vi "Add to Array.vi"(8 "error in (no error)":errorcluster, 9 "Module?":bool, 10 "Position Index":dbl, 11 "Database Entry in":refnum<class "Database Entry.lvclass">) -> (0 "error out":errorcluster, 3 "Database Entry out":refnum<class "Database Entry.lvclass">)   [LabVIEW 2021, in "Database Entry.lvclass"]
uses:
  Database Entry.lvclass
  Stack/Stack.lvclass
  Database Entry.lvclass/Database Entry.ctl
panel:
  out "Array":dbl[](array[numeric])
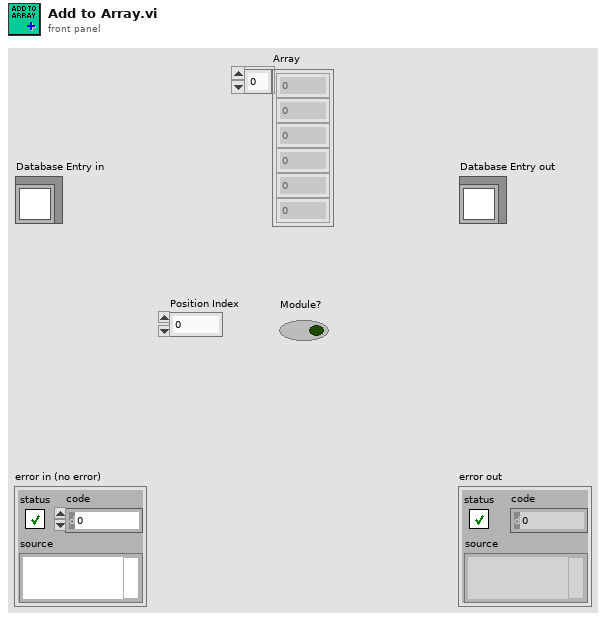
[diagram p1: front panel]
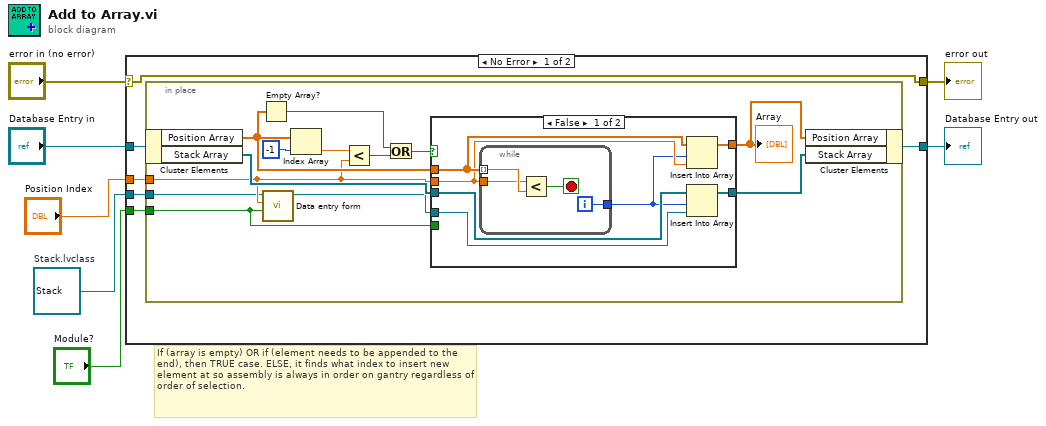
[diagram p0: block diagram]
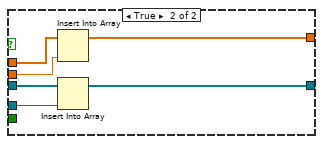
[diagram p2: hidden frame]
diagram:
  w2 = refnum<class "Stack.lvclass"> refnum  # Stack.lvclass
  # "If (array is empty) OR if (element needs to be appended to the end), then TRUE case. ELSE, it finds what index to insert new element at so assembly is always in order on gantry regardless of order of selection."
  n1 = case shown="No Error" "error in (no error)" {
    selector: "error in (no error)" -> [w13 w45]
    tunnel: [w13 w45] -> w6
    tunnel: [w10 w44] -> w4
    tunnel: "Database Entry in" -> [w11 w44]
    tunnel: w2 -> [w12 _]
    tunnel: "Position Index" -> [w9 _]
    tunnel: "Module?" -> [w8 _]
    frame No Error {
      n2 = in-place {
        in-place-border: w12 -> [w14]
        in-place-border: w9 -> [w16]
        in-place-border: w8 -> [w15]
        n3 = in-place-cluster #1(w11) -> ("Position Array"=w23:dbl[], "Stack Array"=w26:refnum<class "Stack.lvclass">[])
        n4 = Empty Array?(array=w23) -> (empty?=w20:bool)
        n5 = call "Data entry form.vi"("Module?"=w15, "Position"=w16, "Stack in"=w14) -> ("Stack out"=w17:refnum<class "Stack.lvclass">)  [unwired: 7 in, 1 out]
        n6 = Index Array(array=w23, index=-1) -> (element=w21:dbl)
        n7 = Less?(x=w21, y=w16) -> (x < y?=w19:bool)
        n8 = Or(x=w20, y=w19) -> (x .or. y?=w18:bool)
        n9 = case shown="False" w18 {
          tunnel: w26 -> [w31 w41]
          tunnel: [w32 w40] -> w25
          tunnel: [w33 w43] -> w24
          tunnel: w15 -> [_ _]
          tunnel: w16 -> [w28 w39]
          tunnel: w23 -> [w29 w42]
          tunnel: w17 -> [w30 w38]
          frame False {
            n10 = while {
              tunnel: w29 -> [w37] mode=indexing
              tunnel: w28 -> [w36]
              tunnel: [w34] -> w27
              i -> [w34]
              stop <- w35 stop-if-true
              n11 = Less?(x=w36, y=w37) -> (x < y?=w35:bool)
            }
            n12 = Insert Into Array(array=w29, index=w27, new element=w28) -> (w33:dbl[])
            n13 = Insert Into Array(array=w31, index=w27, new element=w30) -> (w32:refnum<class "Stack.lvclass">[])
          }
          frame True {
            n14 = Insert Into Array(array=w42, new element=w39) -> (w43:dbl[])  [unwired: 1 in]
            n15 = Insert Into Array(array=w41, new element=w38) -> (w40:refnum<class "Stack.lvclass">[])  [unwired: 1 in]
          }
        }
        "Array" <- w24
        n16 = in-place-cluster #1("Position Array"=w24, "Stack Array"=w25) -> (w10:refnum<class "Database Entry.lvclass">)
      }
    }
    frame Error {
    }
  }
  "error out" <- w6
  "Database Entry out" <- w4
